vi "TEMPConfigure Dialog.vi"(8 "error in (no error)":errorcluster, 11 "Message in":refnum<class "Message.lvclass">) -> (0 "error out":errorcluster, 2 "Ok?":bool, 3 "Message out":refnum<class "Message.lvclass">)   [LabVIEW 2016, in "AsynchReturnDialog Template.lvclass"]
uses:
  AsynchReturnDialog Template.lvclass
  <vilib>/ActorFramework/Message/Message.lvclass
  <vilib>/ActorFramework/Actor/Actor.lvclass
panel:
  in  "Cancel Button":bool
  in  "OK Button":bool
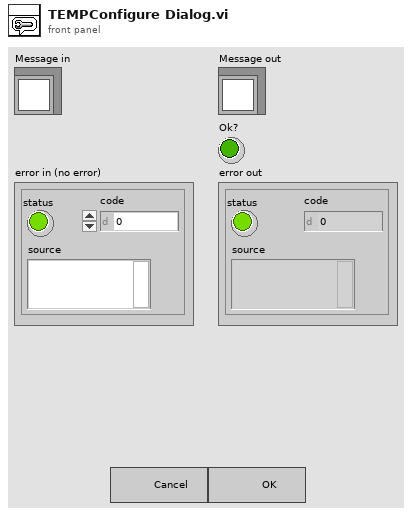
[diagram p1: front panel]
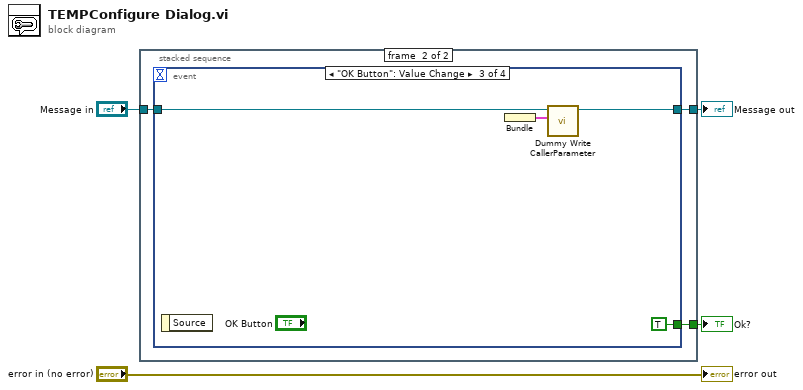
[diagram p0: block diagram]
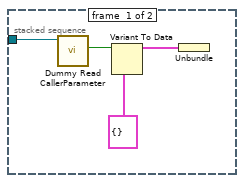
[diagram p2: hidden frame]
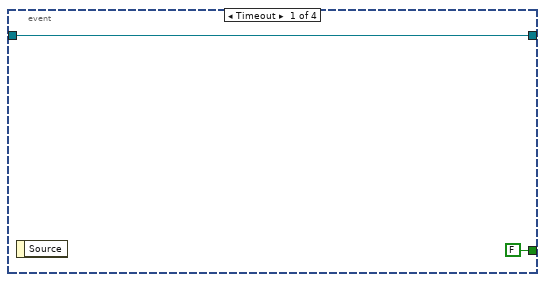
[diagram p3: hidden frame]
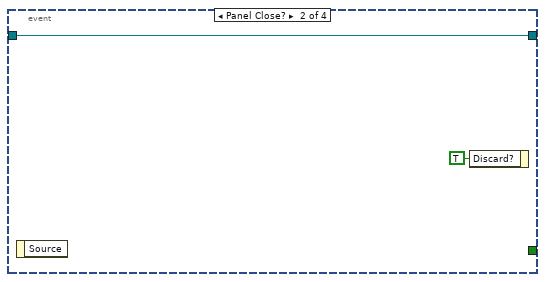
[diagram p4: hidden frame]
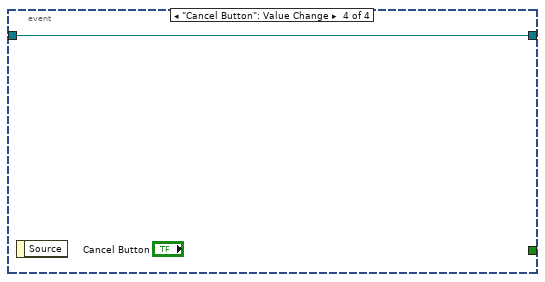
[diagram p5: hidden frame]
diagram:
  n1 = stacked-sequence {
    tunnel: [_ w11] -> w3
    tunnel: [_ w10] -> w2
    tunnel: "Message in" -> [w8 w9]
    frame #0 {
      n2 = call "Dummy Read CallerParameter.vi"("Actor in"=w8) -> ("Boolean"=w7:bool)  [unwired: 8 in, 2 out]
      n3 = Variant To Data(type=cluster{} {} ("Type"), Variant=w7) -> (data=w6:cluster{})  [unwired: 1 in, 1 out]
      n4 = Unbundle ("Seq0Unbundler")(w6) -> ()  [unwired: 1 out]
    }
    frame #1 {
      n5 = event shown="[2] \"OK Button\": Value Change" {
        selector: _ -> [_ _ _ _]
        dyn-events: _ -> [_ _ _ _]
        timeout: _ -> [_ _ _ _]
        tunnel: [w12 w14 w17 w20] -> w10
        tunnel: w9 -> [w12 w14 w16 w20]
        tunnel: [FALSE _ TRUE _] -> w11
        event Timeout {
          n6 = event-data() -> ()  [unwired: 1 in, 1 out]
        }
        event Panel Close? {
          n7 = event-data() -> ()  [unwired: 1 in, 1 out]
          n8 = event-data("Discard?"=TRUE) -> ()  [unwired: 1 in, 1 out]
        }
        event "OK Button": Value Change {
          n9 = event-data() -> ()  [unwired: 1 in, 1 out]
          n10 = Bundle ("Main-Bundler")() -> (w18:cluster{void})  [unwired: 2 in]
          n11 = call "Dummy Write CallerParameter.vi"("Boolean"=w18, "Actor in"=w16) -> ("Actor out"=w17:refnum<class "Actor.lvclass">)  [unwired: 7 in, 1 out]
        }
        event "Cancel Button": Value Change {
          n12 = event-data() -> ()  [unwired: 1 in, 1 out]
        }
      }
    }
  }
  "Ok?" <- w3
  "Message out" <- w2
  "error out" <- "error in (no error)"
